vi "Create Optimiser SBlock.vi"(8 "error in (no error)":errorcluster, 11 "Schedule Block in":refnum<class "Schedule Block.lvclass">) -> (0 "error out":errorcluster, 3 "Optimiser SBlock out":refnum<class "Optimiser SBlock.lvclass">)   [LabVIEW 2020, in "TALOS.lvlib" / "Run Utilities.lvlib" / "Optimiser SBlock.lvclass"]
uses:
  Optimiser SBlock.lvclass
  C:/LabVIEW Code/TALOS/talos/Run Utilities/Schedule Block/Schedule Block.lvclass
  Schedule Block/Schedule Block.lvclass
  Schedule/Schedule.lvclass
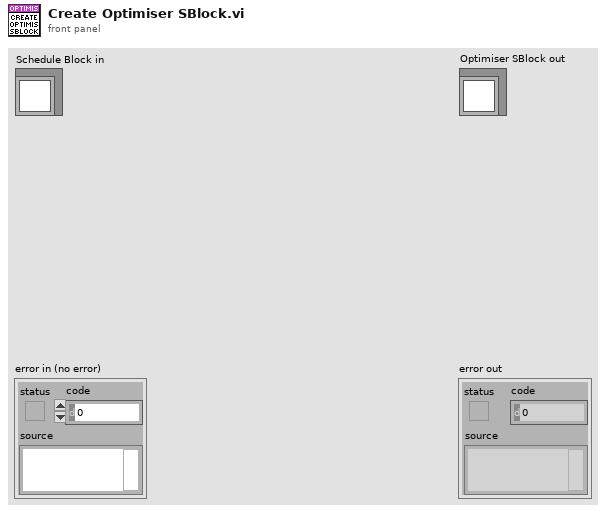
[diagram p1: front panel]
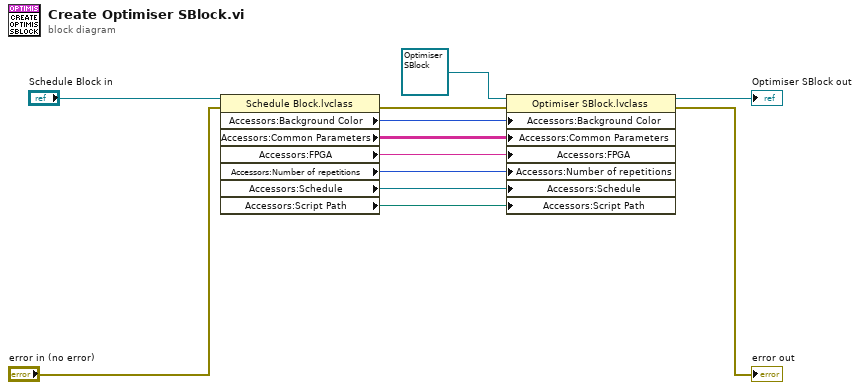
[diagram p0: block diagram]
diagram:
  n1 = property class="Schedule Block.lvclass"(reference="Schedule Block in", error in="error in (no error)") -> (error out=w11:errorcluster, "Accessors:Background Color"=w10:u32, "Accessors:Common Parameters"=w9:string[][], "Accessors:FPGA"=w8:string, "Accessors:Number of repetitions"=w7:u16, "Accessors:Schedule"=w6:refnum<class "Schedule.lvclass">, "Accessors:Script Path"=w5:path)  [unwired: 1 out]
  n2 = property class="Optimiser SBlock.lvclass"(reference=refnum<class "Optimiser SBlock.lvclass"> refnum ("Optimiser SBlock out"), error in=w11, "Accessors:Background Color"=w10, "Accessors:Common Parameters"=w9, "Accessors:FPGA"=w8, "Accessors:Number of repetitions"=w7, "Accessors:Schedule"=w6, "Accessors:Script Path"=w5) -> (reference out=→"Optimiser SBlock out":refnum<class "Optimiser SBlock.lvclass">, error out=→"error out":errorcluster)
